vi "Update Protection Signals.vi"(8 "error in (no error)":errorcluster, 9 "Overrides":dbl[](array[numeric]), 10 "Protections":T1, 11 "Frame Settings in":T2 {"Protection Configurations"."CRC Channels"."Data Type" items=["Signed", "Unsigned", "IEEE Float"]}) -> (0 "error out":errorcluster, 3 "Frame Settings out":T2 {"Protection Configurations"."CRC Channels"."Data Type" items=["Signed", "Unsigned", "IEEE Float"]})   [LabVIEW 2024, in "Protection and Counter Support Engine.lvlib"]
uses:
  Protection and Counter Support Engine.lvlib
  Types/RT Frame Settings.ctl
  Shared/Types/Exported Frame Type.ctl
  Types/RT Protection Configuration.ctl
  Shared/Types/Protection Type.ctl
  Shared/Types/XNET Signal Configuration.ctl
  Shared/Types/Exported Counter Settings.ctl
  Shared/Types/Exported Event Trigger Type.ctl
  <vilib>/NI/NIVS Inline Async API/_Data Access Engine/Data Access Engine/Types/Write.DVR.ctl
  <vilib>/NI/NIVS Inline Async API/_Data Access Engine/Access Type Classes/Write/Write.lvclass
  <vilib>/NI/NIVS Inline Async API/_Data Access Engine/Access Type Classes/Write/Write.lvclass/Write.ctl
  <vilib>/NI/NIVS Inline Async API/_Data Access Engine/Data Access Engine/Methods/Data.Processes.Execute.vi
  <vilib>/NI/NIVS Inline Async API/_Data Access Engine/Data Access Engine/Methods/Write.Data.Buffer.vi
  Get Protection Signals.vi
  <vilib>/NI/NIVS Inline Async API/_Data Access Engine/Access Type Classes/Write/Write.Buffer.vi
  <vilib>/xnet/xnet.llb/XNET Convert.vi
  <vilib>/xnet/xnet.llb/XNET Convert (Signal to Frame Raw).vi
  Shared/Protection and Counter Support Shared.lvlib
  <vilib>/NI/NIVS Inline Async API/_Data Access Engine/Data Access Engine/Data Access Engine.lvclass
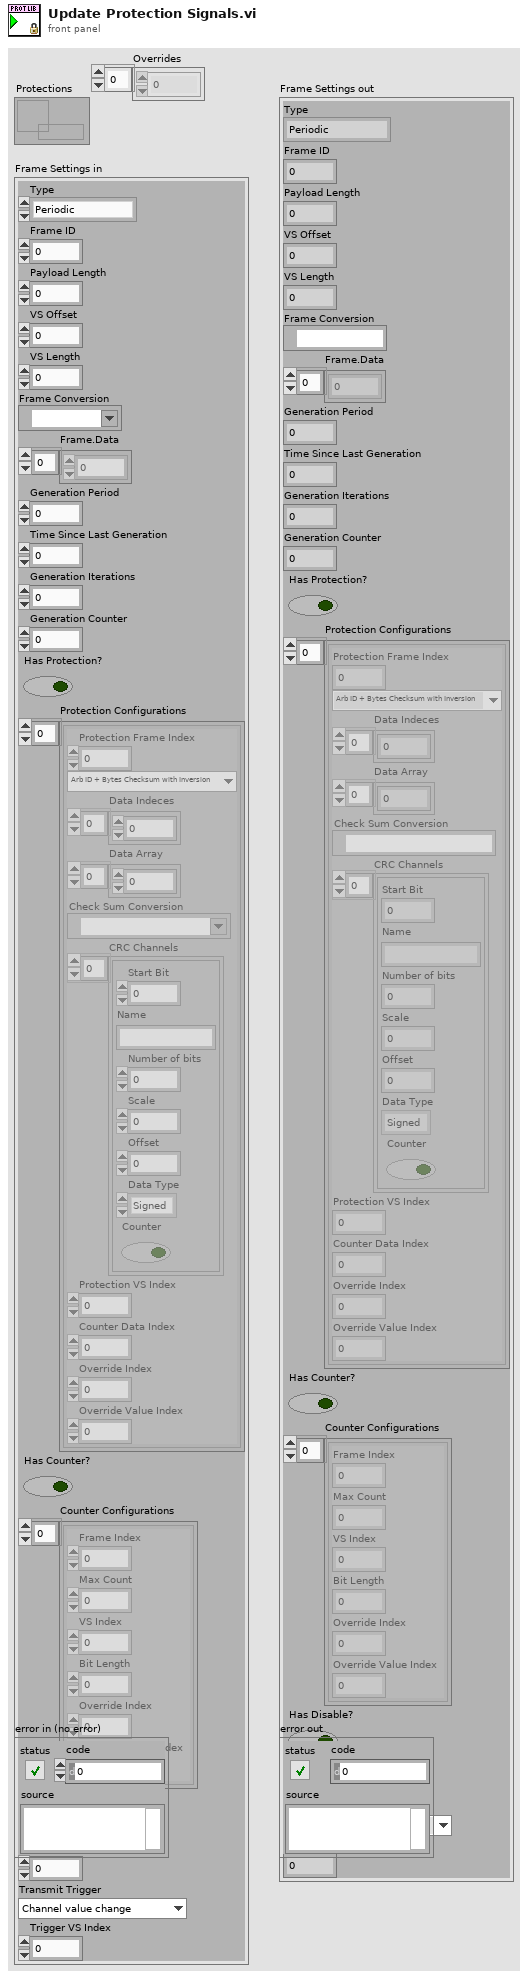
[diagram p1: front panel]
types:
  T1 = typedef "Data Access Engine.lvlib/Data Access Engine.lvclass/Write.DVR.ctl" = refnum<data-value>
  T2 = typedef "Protection and Counter Support Engine.lvlib/RT Frame Settings.ctl" = cluster{"Type":T3, "Frame ID":u32, "Payload Length":u32, "VS Offset":i32, "VS Length":i32, "Frame Conversion":refnum<k21>, "Frame.Data":dbl[], "Generation Period":u32, "Time Since Last Generation":u32, "Generation Iterations":u32, "Generation Counter":u32, "Has Protection?":bool, "Protection Configurations":T4[], "Has Counter?":bool, "Counter Configurations":T7[], "Has Disable?":bool, "Disable VS Index":i32, "Transmit Trigger":T8, "Trigger VS Index":i32}
  T3 = typedef "Protection and Counter Support Shared.lvlib/Exported Frame Type.ctl" = enum16{"Periodic", "Event", "Periodic/Event"}
  T4 = typedef "Protection and Counter Support Engine.lvlib/RT Protection Configuration.ctl" = cluster{"Protection Frame Index":i32, "Protection Type":T5, "Data Indeces":i32[], "Data Array":dbl[], "Check Sum Conversion":refnum<k21>, "CRC Channels":T6[], "Protection VS Index":i32, "Counter Data Index":i32, "Override Index":i32, "Override Value Index":i32}
  T5 = typedef "Protection and Counter Support Shared.lvlib/Protection Type.ctl" = enum16{"Arb ID + Bytes Checksum with Inversion", "Arb ID + Bytes CRC with Inversion", "Reversed Raw Signal Checksum with Inversion", "Concatenated Two's Compliment"}
  T6 = typedef "Protection and Counter Support Shared.lvlib/XNET Signal Configuration.ctl" = cluster{"Start Bit":i32, "Name":string, "Number of bits":i32, "Scale":dbl, "Offset":dbl, "Data Type":u32, "Counter":bool}
  T7 = typedef "Protection and Counter Support Shared.lvlib/Exported Counter Settings.ctl" = cluster{"Frame Index":i32, "Max Count":dbl, "VS Index":i32, "Bit Length":i64, "Override Index":i32, "Override Value Index":i32}
  T8 = typedef "Protection and Counter Support Shared.lvlib/Exported Event Trigger Type.ctl" = enum16{"Channel value change", "Trigger channel (not zero)", "Channel value change or trigger channel (not zero)", "Trigger channel (any value change)", "Channel value change or trigger channel (any value change)"}
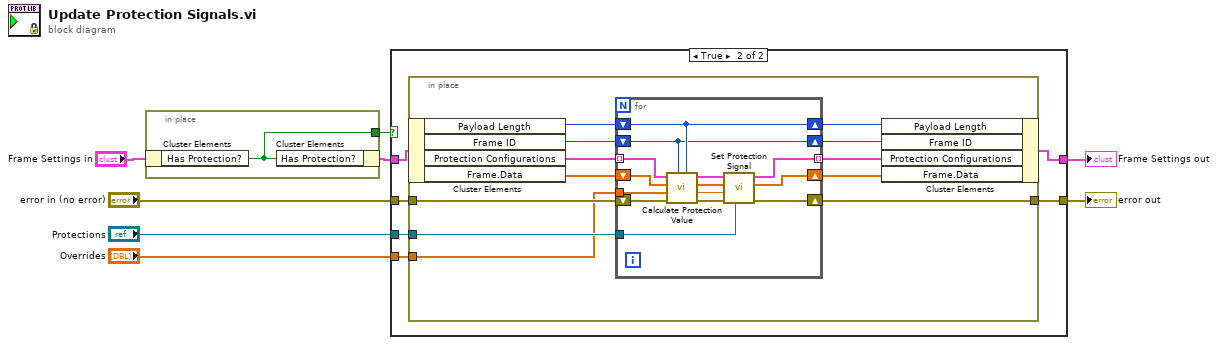
[diagram p0: block diagram]
diagram:
  n1 = in-place {
    in-place-border: [w9] -> w3
    n2 = in-place-cluster #1("Frame Settings in") -> ("Has Protection?"=w9:bool)
    n3 = in-place-cluster #1("Has Protection?"=w9) -> (w2:T2)
  }
  n4 = case shown="True" w3 {
    tunnel: "error in (no error)" -> [w11 w17]
    tunnel: [w11 w16] -> w5
    tunnel: "Protections" -> [_ w15]
    tunnel: [w10 w13] -> w8
    tunnel: w2 -> [w10 w14]
    tunnel: "Overrides" -> [_ w12]
    frame False {
    }
    frame True {
      n5 = in-place {
        in-place-border: w17 -> [w29]
        in-place-border: [w28] -> w16
        in-place-border: w15 -> [w27]
        in-place-border: w12 -> [w18]
        n6 = in-place-cluster #2(w14) -> ("Payload Length"=w24:u32, "Frame ID"=w23:u32, "Protection Configurations"=w20:T4[], "Frame.Data"=w26:dbl[])
        n7 = for {
          tunnel: w20 -> [w35] mode=indexing
          shift-right: [w39] -> w28
          shift-left: w29 -> [w43]
          shift-right: [w32] -> w25
          shift-left: w26 -> [w34]
          tunnel: w27 -> [w31]
          tunnel: [w36] -> w19 mode=indexing
          shift-right: [w42] -> w22
          shift-left: w24 -> [w42]
          shift-right: [w41] -> w21
          shift-left: w23 -> [w41]
          tunnel: w18 -> [w30]
          n8 = call "Calculate Protection Value.vi"("Payload Length"=w42, "Frame ID"=w41, "error in (no error)"=w43, "Overrides"=w30, "Frame.Data in"=w34, "Protection Configuration in"=w35) -> ("error out"=w40:errorcluster, "Protection Value"=w33:dbl, "Frame.Data out"=w37:dbl[], "Protection Configuration out"=w38:T4)  [unwired: 2 in]
          n9 = call "Set Protection Signal.vi"("Protections"=w31, "error in (no error)"=w40, "Protection Value"=w33, "Frame.Data in"=w37, "Protection Configuration in"=w38) -> ("error out"=w39:errorcluster, "Frame.Data out"=w32:dbl[], "Protection Configuration out"=w36:T4)  [unwired: 4 in]
        }
        n10 = in-place-cluster #2("Payload Length"=w22, "Frame ID"=w21, "Protection Configurations"=w19, "Frame.Data"=w25) -> (w13:T2)
      }
    }
  }
  "Frame Settings out" <- w8
  "error out" <- w5
